vi "Get Target IP and Name.vi"(8 "error in (no error)":errorcluster, 11 "Item Ref in":T1 format="%.0x") -> (0 "error out":errorcluster, 1 "Name":string, 2 "IPAddress":string, 3 "Item Ref out":T1=18446744073709551615 format="%.0x")   [LabVIEW 2015, in "Diagnostics Addon System Explorer.lvlib"]
uses:
  Diagnostics Addon System Explorer.lvlib
  <vilib>/NI Veristand/Custom Device API/Custom Device Item Ref.ctl
  NationalInstruments.VeriStand.SystemDefinitionAPI
  <vilib>/NI Veristand/Custom Device Offline API/Custom Device Offline API.lvlib
  <vilib>/NI Veristand/Custom Device Tools/Custom Device Utility Library/Custom Device Utility Library.lvlib
  <vilib>/NI Veristand/Custom Device API/Custom Device API.lvlib
panel:
  # "OUTPUTS"
  # "INPUTS"
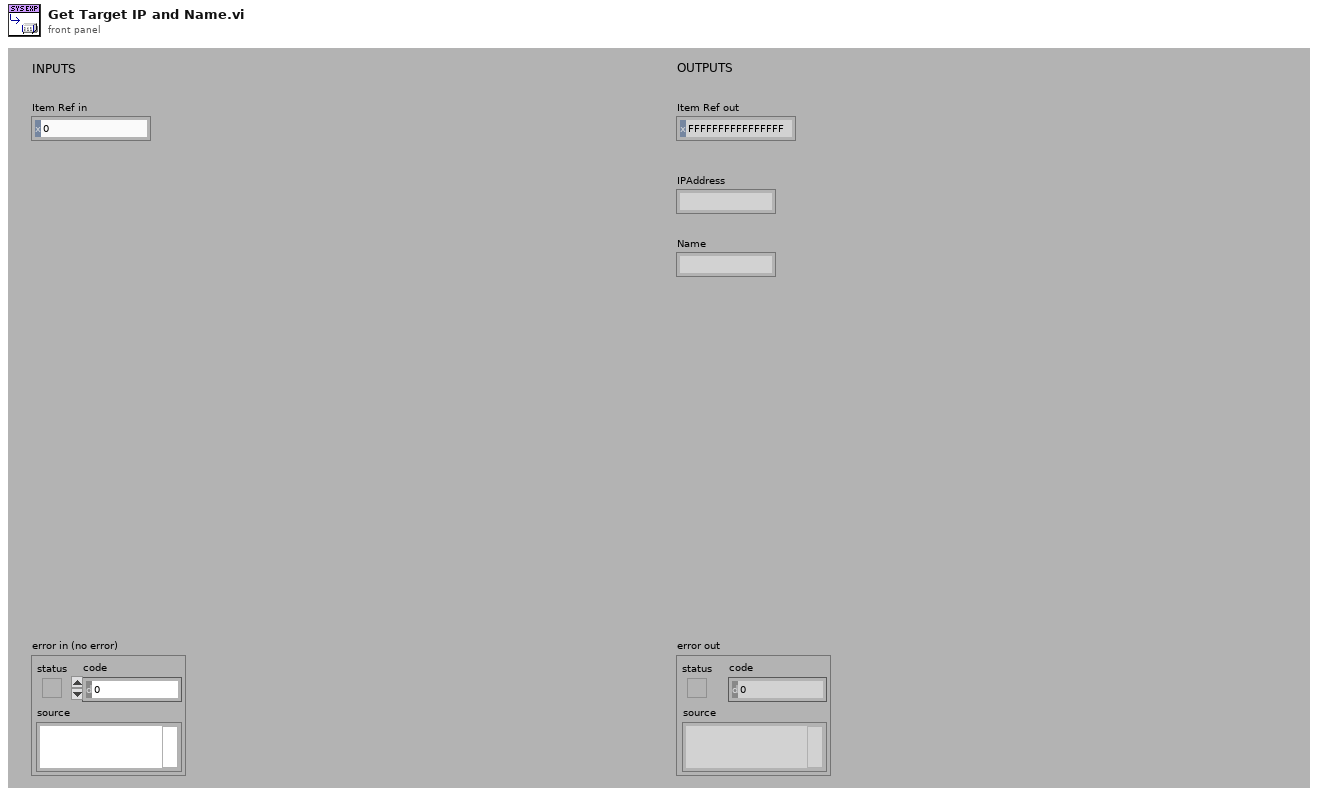
[diagram p1: front panel]
types:
  T1 = typedef "Custom Device API.lvlib/Custom Device Item Ref.ctl" = u64
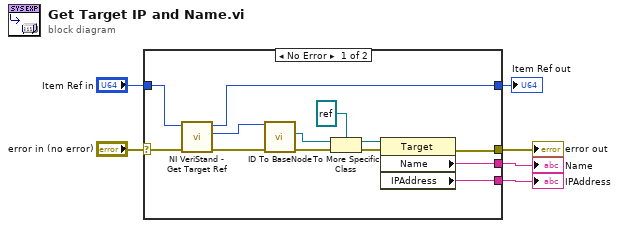
[diagram p0: block diagram]
diagram:
  n1 = case shown="No Error" "error in (no error)" {
    selector: "error in (no error)" -> [w16 w21]
    tunnel: [w10 w21] -> w5
    tunnel: "Item Ref in" -> [w17 w20]
    tunnel: [w9 _] -> w3
    tunnel: [w8 _] -> w2
    tunnel: [w7 w20] -> w1
    frame No Error {
      n2 = call <vilib>:"NI VeriStand - Get Target Ref.vi"("error in"=w16, "Item Ref in"=w17) -> ("error out"=w18:errorcluster, "Target Ref"=w19:T1, "Item Ref out"=w7:T1)  [unwired: 6 in, 1 out]
      n3 = call <vilib>:"ID To BaseNode.vi"("error in (no error)"=w18, "ID in"=w19) -> ("error out"=w11:errorcluster, "BaseNode"=w12:refnum<k24>)  [unwired: 7 in, 1 out]
      n4 = To More Specific Class(target class=refnum<k24> refnum, reference=w12, error in=w11) -> (specific class reference=w14:refnum<k24>, error out=w15:errorcluster)
      n5 = property class="Target"(reference=w14, error in=w15) -> (error out=w10:errorcluster, "Name"=w9:string, "IPAddress"=w8:string)  [unwired: 1 out]
    }
    frame Error {
    }
  }
  "error out" <- w5
  "Name" <- w3
  "IPAddress" <- w2
  "Item Ref out" <- w1
